vi "Show Window.vi"(8 "error in":errorcluster caption="error in (no error)" {"code" format="%d\n%x"}, 10 "window name (\"\")":string, 11 "window refnum":T1 caption="window refnum (NaWR)") -> (0 "error out":errorcluster {"code" format="%d\n%x"}, 3 "window refnum out":T1)   [LabVIEW 2020, in "Win Util New.lvlib"]
doc: "This function will show a previously hidden window. The window named in the 'window name' input is used to identify the target window if 'window refnum' is invalid. If the window cannot be found, an error will be returned and 'window refnum out' will be invalid."
uses:
  Win Util New.lvlib
  Window Refnum.ctl
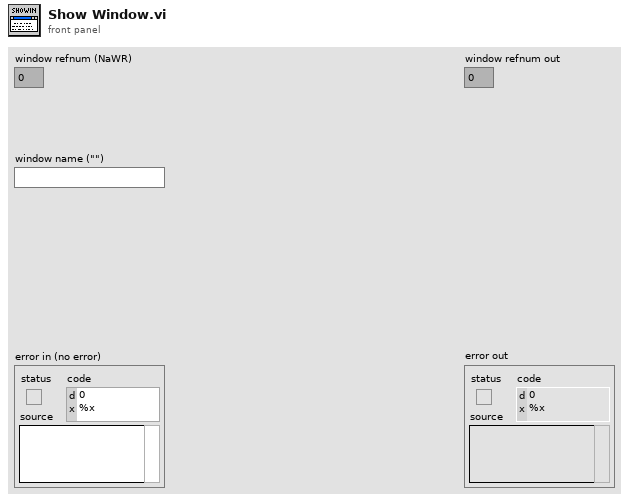
[diagram p1: front panel]
types:
  T1 = typedef "Win Util New.lvlib/Window Refnum.ctl" = u64
  T2 = enum8{"SW_HIDE", "SW_SHOWNORMAL", "SW_SHOWMINIMIZED", "SW_MAXIMIZE", "SW_SHOWNOACTIVATE", "SW_SHOW", "SW_MINIMIZE", "SW_SHOWMINNOACTIVATE", "SW_SHOWNA", "SW_RESTORE", "SW_SHOWDEFAULT", "SW_FORCEMINIMIZE"}
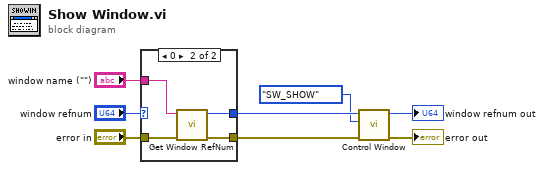
[diagram p0: block diagram]
diagram:
  n1 = case shown="0" "window refnum" {
    selector: "window refnum" -> [w9 _]
    tunnel: "error in" -> [w10 w14]
    tunnel: [w9 w13] -> w4
    tunnel: [w10 w12] -> w5
    tunnel: "window name (\"\")" -> [_ w11]
    frame Default {
    }
    frame 0 {
      n2 = call "Get Window RefNum.vi"("error in"=w14, "window name (\"\")"=w11) -> ("error out"=w12:errorcluster, "window refnum (NaWR)"=w13:T1)  [unwired: 6 out]
    }
  }
  n3 = call "Control Window.vi"("error in"=w5, "Function"=T2."SW_SHOW" ("function"), "window refnum"=w4) -> ("error out"=→"error out":errorcluster, "dup window refnum"=→"window refnum out":T1)  [unwired: 7 in]
